vi "FooterGUI.vi"() -> ()   [LabVIEW 2021, in "FooterTriekselSoft.lvclass"]
uses:
  FooterTriekselSoft.lvclass
panel:
  out "String":string
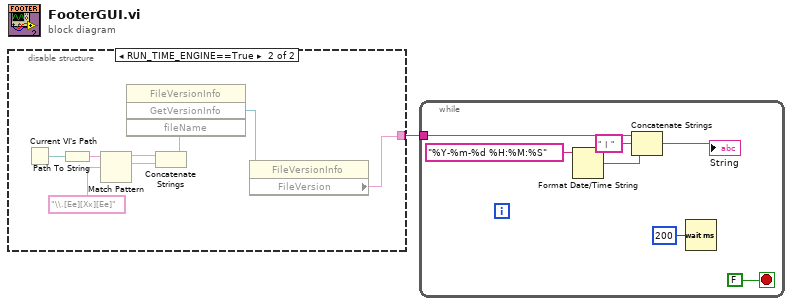
[diagram p0: block diagram]
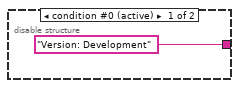
[diagram p2: hidden frame]
diagram:
  n1 = disable-structure shown="RUN_TIME_ENGINE==True" {
    disable-tunnel: ["Version: Development" w3] -> w1
    frame condition #0 (active) {
    }
    frame condition #1 {
      n2 = Current VI's Path() -> (path=w6:path)
      n3 = Path To String(path=w6) -> (string=w10:string)
      n4 = Match Pattern(string=w10, regular expression="\\.[Ee][Xx][Ee]") -> (before substring=w8:string, match substring=w7:string)  [unwired: 1 in, 2 out]
      n5 = Concatenate Strings(w8, w7) -> (w9:string)
      n6 = invoke class="FileVersionInfo" method="GetVersionInfo"("fileName"=w9) -> ("GetVersionInfo"=w5:refnum<k24>)  [unwired: 3 in, 3 out]
      n7 = property class="FileVersionInfo"(reference=w5) -> ("FileVersion"=w3:string)  [unwired: 1 in, 2 out]
    }
  }
  n8 = while {
    tunnel: w1 -> [w13]
    stop <- FALSE stop-if-true
    n9 = Format Date/Time String(time format string (%c)="%Y-%m-%d %H:%M:%S") -> (date/time string=w14:string)  [unwired: 2 in]
    n10 = Concatenate Strings(w13, "  |  " ("string"), w14) -> (→"String":string)
    n11 = Wait (ms)(milliseconds to wait=u32 200) -> ()  [unwired: 1 out]
  }
